vi "Connect.vi"(8 "error in":errorcluster, 11 "Control Box in":refnum<class "Control Box.lvclass">) -> (0 "error out":errorcluster, 3 "Control Box out":refnum<class "Control Box.lvclass">)   [LabVIEW 2018, in "Control Box.lvlib" / "Control Box.lvclass"]
uses:
  Control Box.lvclass
  Control Box.lvclass/Control Box.ctl
  <vilib>/Instr/_visa.llb/VISA Configure Serial Port (Instr).vi
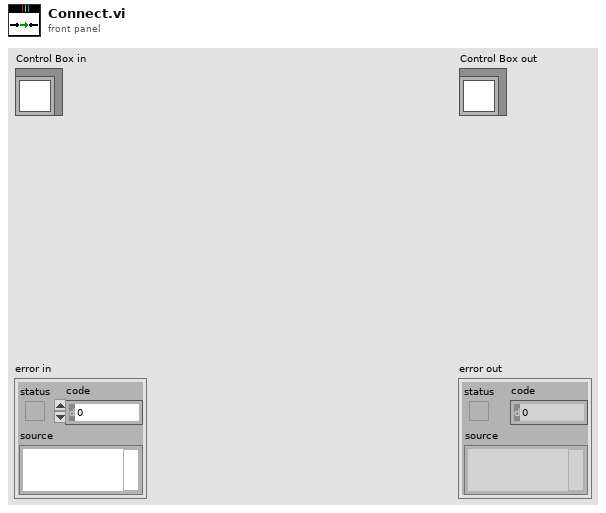
[diagram p1: front panel]
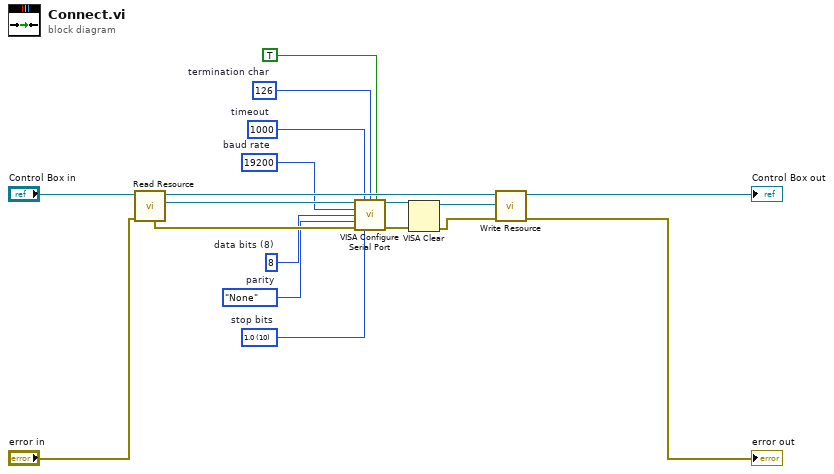
[diagram p0: block diagram]
diagram:
  w1 = u16 10 items=["1.0"=10, "1.5"=15, "2.0"=20]  # stop bits
  w2 = enum16{"None", "Odd", "Even", "Mark", "Space"}."None"  # parity
  w3 = u16 8  # data bits (8)
  w4 = u32 19200  # baud rate
  w5 = u32 1000  # timeout
  w6 = u8 126  # termination char
  n1 = call "Read Resource.vi"("error in (no error)"="error in", "Control Box in"="Control Box in") -> ("error out"=w14:errorcluster, "Resource"=w17:refnum<visa-resource-name>, "Control Box out"=w13:refnum<class "Control Box.lvclass">)  [unwired: 7 in]
  n2 = call-poly "VISA Configure Serial Port"("VISA resource name"=w17, "timeout (10sec)"=w5, "termination char\n(0xA = '\\n' = LF)"=w6, "Enable Termination\nChar (T)"=TRUE ("Enable Termination\nChar (T)"), "baud rate (9600)"=w4, "data bits (8)"=w3, "parity (0:none)"=w2, "error in (no error)"=w14, "stop bits (10: 1 bit)"=w1) -> ("VISA resource name out"=w15:refnum<visa-resource-name>, "error out"=w16:errorcluster)  [unwired: 5 in]
  n3 = VISA Clear(VISA resource name=w15, error in (no error)=w16) -> (VISA resource name out=w11:refnum<visa-resource-name>, error out=w10:errorcluster)
  n4 = call "Write Resource.vi"("error in (no error)"=w10, "Resource"=w11, "Control Box in"=w13) -> ("error out"=→"error out":errorcluster, "Control Box out"=→"Control Box out":refnum<class "Control Box.lvclass">)  [unwired: 7 in]
